vi "Pump 2 Sub.vi"(7 "P2 Direction":bool=TRUE, 8 "Error In":errorcluster, 9 "P2 pps":dbl=100.0, 10 "P2 Steps":u32=250, 11 "FPGA ref in":refnum<k20>) -> (0 "Error out":errorcluster, 3 "FPGA ref out":refnum<k20>)   [LabVIEW 2013]
uses:
  <vilib>/rvi/interface/common/niFpgaWaitOnOcc.vi
  <vilib>/Utility/error.llb/Error Cluster From Error Code.vi
  <vilib>/rvi/errors/niLvFpgaAdjustHostInterfaceError.vi
  <vilib>/rvi/interface/nirviReadWriteControl/nirviReadWriteControl.xnode
  <vilib>/rvi/interface/Simulation/niFpgaSimulationCallBeginRW.vi
  NiFpgaLv.dll
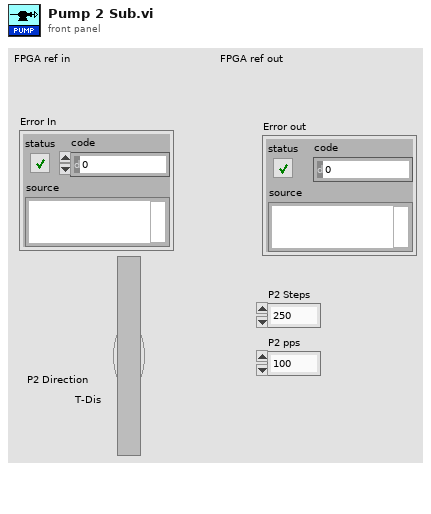
[diagram p1: front panel]
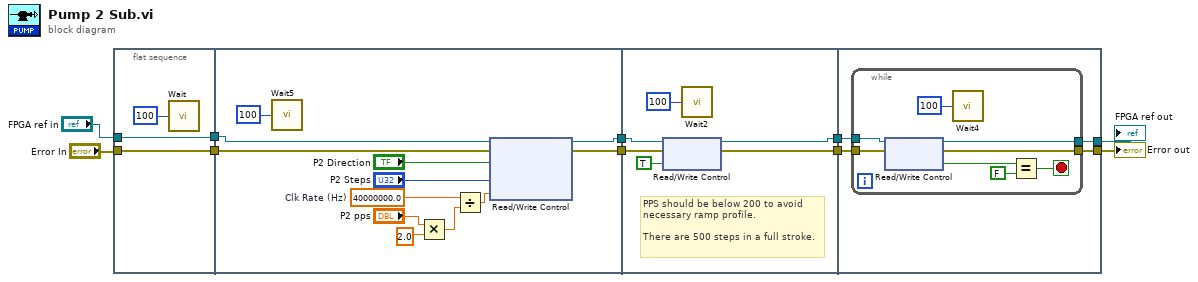
[diagram p0: block diagram]
diagram:
  n1 = flat-sequence {
    tunnel: "Error In" -> [w13]
    tunnel: [w13] -> w7
    tunnel: [w11] -> w3
    tunnel: "FPGA ref in" -> [w11]
    tunnel: [w24] -> w8
    tunnel: w7 -> [w22]
    tunnel: [w25] -> w6
    tunnel: w3 -> [w14]
    tunnel: [w28] -> w9
    tunnel: [w27] -> w10
    tunnel: w8 -> [w30]
    tunnel: w6 -> [w29]
    tunnel: w10 -> [w35]
    tunnel: w9 -> [w34]
    tunnel: [w33] -> w1
    tunnel: [w32] -> w5
    frame #0 {
      n2 = call "Wait"("Count(mSec)"=u32 100) -> ()  [unwired: 1 out]
    }
    frame #1 {
      w20 = 40000000.0  # Clk Rate (Hz)
      n3 = call "Wait5"("Count(mSec)"=u32 100) -> ()  [unwired: 1 out]
      n4 = Multiply(x="P2 pps", y=2.0) -> (x*y=w16:dbl)
      n5 = Divide(x=w20, y=w16) -> (x/y=w17:dbl)
      n6 = xnode "Read/Write Control"("FPGA VI Reference In"=w14, "error in"=w22, "P2 Direction"="P2 Direction", "P2 Steps"="P2 Steps", "P2 Period"=w17) -> ("FPGA VI Reference Out"=w24:refnum<k20>, "error out"=w25:errorcluster)
    }
    frame #2 {
      # "PPS should be below 200 to avoid \nnecessary ramp profile.\n\nThere are 500 steps in a full stroke."
      n7 = xnode "Read/Write Control"("FPGA VI Reference In"=w30, "error in"=w29, "Start P2"=TRUE ("Pump 2 PWR")) -> ("FPGA VI Reference Out"=w27:refnum<k20>, "error out"=w28:errorcluster)
      n8 = call "Wait2"("Count(mSec)"=u32 100) -> ()  [unwired: 1 out]
    }
    frame #3 {
      n9 = while {
        tunnel: w35 -> [w43]
        tunnel: w34 -> [w42]
        tunnel: [w41] -> w33
        tunnel: [w40] -> w32
        stop <- w36 stop-if-true
        n10 = xnode "Read/Write Control"("FPGA VI Reference In"=w43, "error in"=w42) -> ("FPGA VI Reference Out"=w41:refnum<k20>, "error out"=w40:errorcluster, "Start P2"=w38:bool)
        n11 = call "Wait4"("Count(mSec)"=u32 100) -> ()  [unwired: 1 out]
        n12 = Equal?(x=w38, y=FALSE) -> (x = y?=w36:bool)
      }
    }
  }
  "Error out" <- w5
  "FPGA ref out" <- w1
